vi "gfitsio-check-fpixel.vi"(8 "error in (no error)":errorcluster, 10 "fpixel":i32[](array[numeric]), 11 "gfits refnum":T1) -> (0 "error out":errorcluster, 2 "fpixel out":i32[](array[numeric]), 3 "dup gfits refnum":T1)   [LabVIEW 2024, in "gfitsio.lvlib"]
uses:
  gfitsio.lvlib
  gfitsio-refnum.ctl
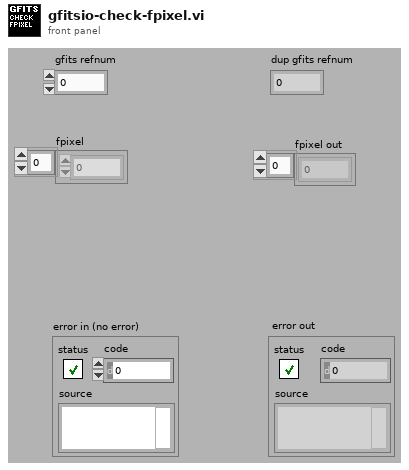
[diagram p1: front panel]
types:
  T1 = typedef "gfitsio.lvlib/gfitsio-refnum.ctl" = u64
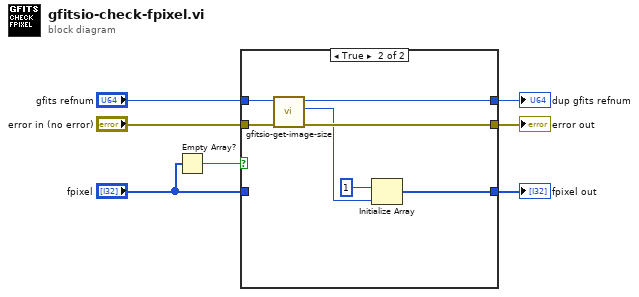
[diagram p0: block diagram]
diagram:
  n1 = Empty Array?(array="fpixel") -> (empty?=w3:bool)
  n2 = case shown="True" w3 {
    tunnel: "error in (no error)" -> [w9 w17]
    tunnel: [w8 w16] -> w6
    tunnel: "gfits refnum" -> [w8 w15]
    tunnel: [w9 w13] -> w4
    tunnel: "fpixel" -> [w10 _]
    tunnel: [w10 w11] -> w1
    frame False {
    }
    frame True {
      n3 = call "gfitsio-get-image-size.vi"("error in (no error)"=w17, "gfits refnum"=w15) -> ("error out"=w13:errorcluster, "naxis"=w12:i32, "dup gfits refnum"=w16:T1)  [unwired: 7 out]
      n4 = Initialize Array(1 ("size(s)"), w12) -> (w11:i32[])
    }
  }
  "error out" <- w4
  "dup gfits refnum" <- w6
  "fpixel out" <- w1
